vi "FTW-SQLite-Backup.vi"(0 "SQLite Connector":refnum<class "FTW-SQLite-Connector.lvclass">, 5 "Destination Database Filepath":path, 11 "error in":errorcluster) -> (4 "SQLite Connector out":refnum<class "FTW-SQLite-Connector.lvclass">, 6 "Time to Execute":dbl format="%.6fsec", 15 "error out":errorcluster)   [LabVIEW 2014, in "FTW-SQLite-Connector.lvclass"]
uses:
  FTW-SQLite-Connector.lvclass
  FTW-SQLite-AccessMode.ctl
  FTW-SQLite-Connector.lvclass/FTW-SQLite-Connector.ctl
  error/FTW-ERR-ThrowGenericError.vi
  error/FTW-ERR-ThrowError.vi
  error/FTW-ERR-CallChain.vi
  string/FTW-STR-ReplaceWhitespace.vi
panel:
  # "Inputs"
  # "Outputs"
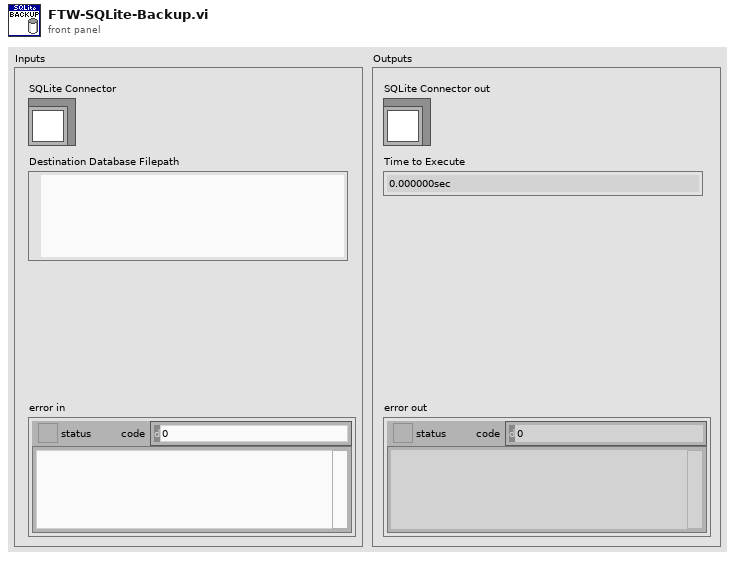
[diagram p1: front panel]
types:
  T1 = typedef "FTW-SQLite-Connector.lvclass/FTW-SQLite-AccessMode.ctl" = enum16{"Read", "Read/Write", "Read/Write/Create"}
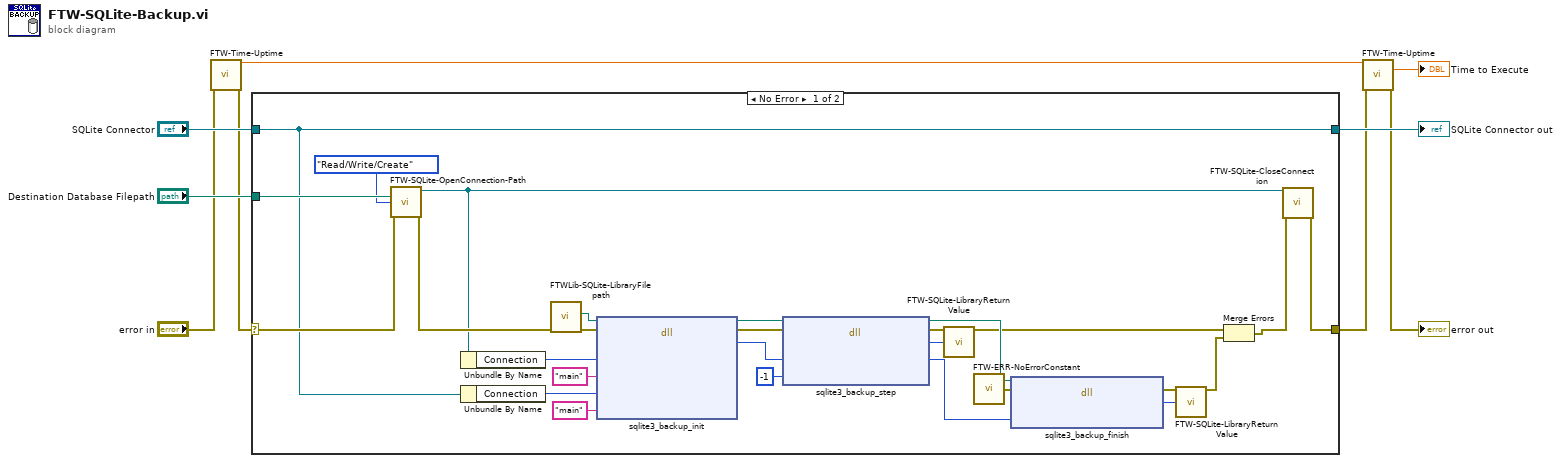
[diagram p0: block diagram]
diagram:
  n1 = call "FTW-Time-Uptime.vi"("error in"="error in") -> ("Current Uptime"=w4:dbl, "error out"=w5:errorcluster)  [unwired: 12 in, 1 out]
  n2 = case shown="No Error" w5 {
    selector: w5 -> [w35 w37]
    tunnel: "SQLite Connector" -> [w24 w38]
    tunnel: [w24 w38] -> w8
    tunnel: "Destination Database Filepath" -> [w36 _]
    tunnel: [w11 w37] -> w2
    frame No Error {
      n3 = call "FTW-SQLite-OpenConnection-Path.vi"("Database Filepath"=w36, "Access Mode"=FTW-SQLite-AccessMode."Read/Write/Create", "error in"=w35) -> ("SQLite Connector"=w13:refnum<class "FTW-SQLite-Connector.lvclass">, "error out"=w34:errorcluster)  [unwired: 11 in]
      n4 = Unbundle By Name(w13) -> ("Connection"=w26:u64)
      n5 = Unbundle By Name(w24) -> ("Connection"=w23:u64)
      n6 = call "FTWLib-SQLite-LibraryFilepath.vi"("error in"=w34) -> ("error out"=w27:errorcluster, "SQLite Library Filepath"=w28:path)  [unwired: 8 in, 1 out]
      n7 = dll-call lib="?" fn="sqlite3_backup_init"(path in=w28, error in=w27, "Destination Pointer"=w26, "Destination Name"="main", "Source Pointer"=w23, "Source Name"="main") -> (path out=w18:path, error out=w15:errorcluster, "Backup Object"=w17:u64)  [unwired: 5 in]
      n8 = dll-call lib="?" fn="sqlite3_backup_step"(path in=w18, error in=w15, "Backup Object"=w17, "NumPages"=-1) -> (path out=w30:path, error out=w21:errorcluster, "Return Type"=w19:i32, "Backup Object"=w33:u64)  [unwired: 2 in]
      n9 = call "FTW-SQLite-LibraryReturnValue.vi"("error in"=w21, "Return Value"=w19) -> ("error out"=w20:errorcluster)  [unwired: 13 in]
      n10 = call "FTW-ERR-NoErrorConstant.vi"() -> ("no error"=w16:errorcluster)
      n11 = dll-call lib="?" fn="sqlite3_backup_finish"(path in=w30, error in=w16, "Backup Object"=w33) -> (error out=w32:errorcluster, "Return Value"=w31:i32)  [unwired: 2 in, 1 out]
      n12 = call "FTW-SQLite-LibraryReturnValue.vi"("error in"=w32, "Return Value"=w31) -> ("error out"=w29:errorcluster)  [unwired: 13 in]
      n13 = Merge Errors(w20, w29) -> (w12:errorcluster)
      n14 = call "FTW-SQLite-CloseConnection.vi"("SQLite Connector"=w13, "error in"=w12) -> ("error out"=w11:errorcluster)  [unwired: 13 in]
    }
    frame Error {
    }
  }
  "SQLite Connector out" <- w8
  n15 = call "FTW-Time-Uptime.vi"("Previous Uptime"=w4, "error in"=w2) -> ("Elapsed Time"=→"Time to Execute":dbl, "error out"=→"error out":errorcluster)  [unwired: 11 in, 1 out]
